vi "G#Object_SendEvent.vi"(0 "reference in":refnum<class "G#Object.lvclass">, 1 "object info extended":T1, 3 "comment":string, 4 "parameters":variant[](array[variant]), 5 "error in (no error)":errorcluster, 6 "G# event type":T3, 7 "send to Desktop Trace Execution":bool=TRUE) -> (19 "error out":errorcluster)   [LabVIEW 2017, in "G#Object.lvclass"]
doc: "Sends object information to the debugger and to the desktop execution trace."
uses:
  G#Object.lvclass
  utils/G#Object_EventType.ctl
  utils/G#Object_ObjectInfoType.ctl
  utils/G#Object_CreateMethod.ctl
  utils/G#Object_Event.ctl
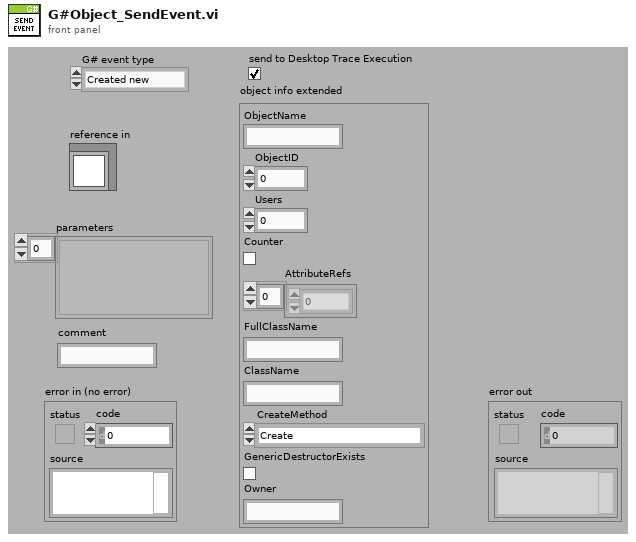
[diagram p1: front panel]
types:
  T1 = typedef "G#Object.lvclass/G#Object_ObjectInfoType.ctl" = cluster{"ObjectName":string, "ObjectID":u32, "Users":i32, "Counter":bool, "AttributeRefs":u32[], "FullClassName":string, "ClassName":string, "CreateMethod":T2, "GenericDestructorExists":bool, "Owner":string}
  T2 = typedef "G#Object.lvclass/G#Object_CreateMethod.ctl" = enum16{"Create", "Create or look up existing", "Look up existing"}
  T3 = typedef "G#Object.lvclass/G#Object_EventType.ctl" = enum16{"Created new", "Looked up existing", "Deleted", "Forced delete", "Not deleted", "Garbage collected", "Cleared", "User", "Error", "External create object", "External create class attributes", "Created class attributes", "Run constructor", "Run constructor done", "Run open method", "Run open method done"}
  T4 = typedef "G#Object.lvclass/G#Object_Event.ctl" = cluster{"EventType":T3, "ObjectInfo":T1, "Ref":refnum<class "G#Object.lvclass">, "Time Stamp":timestamp, "LogText":string, "Parameters":variant[]}
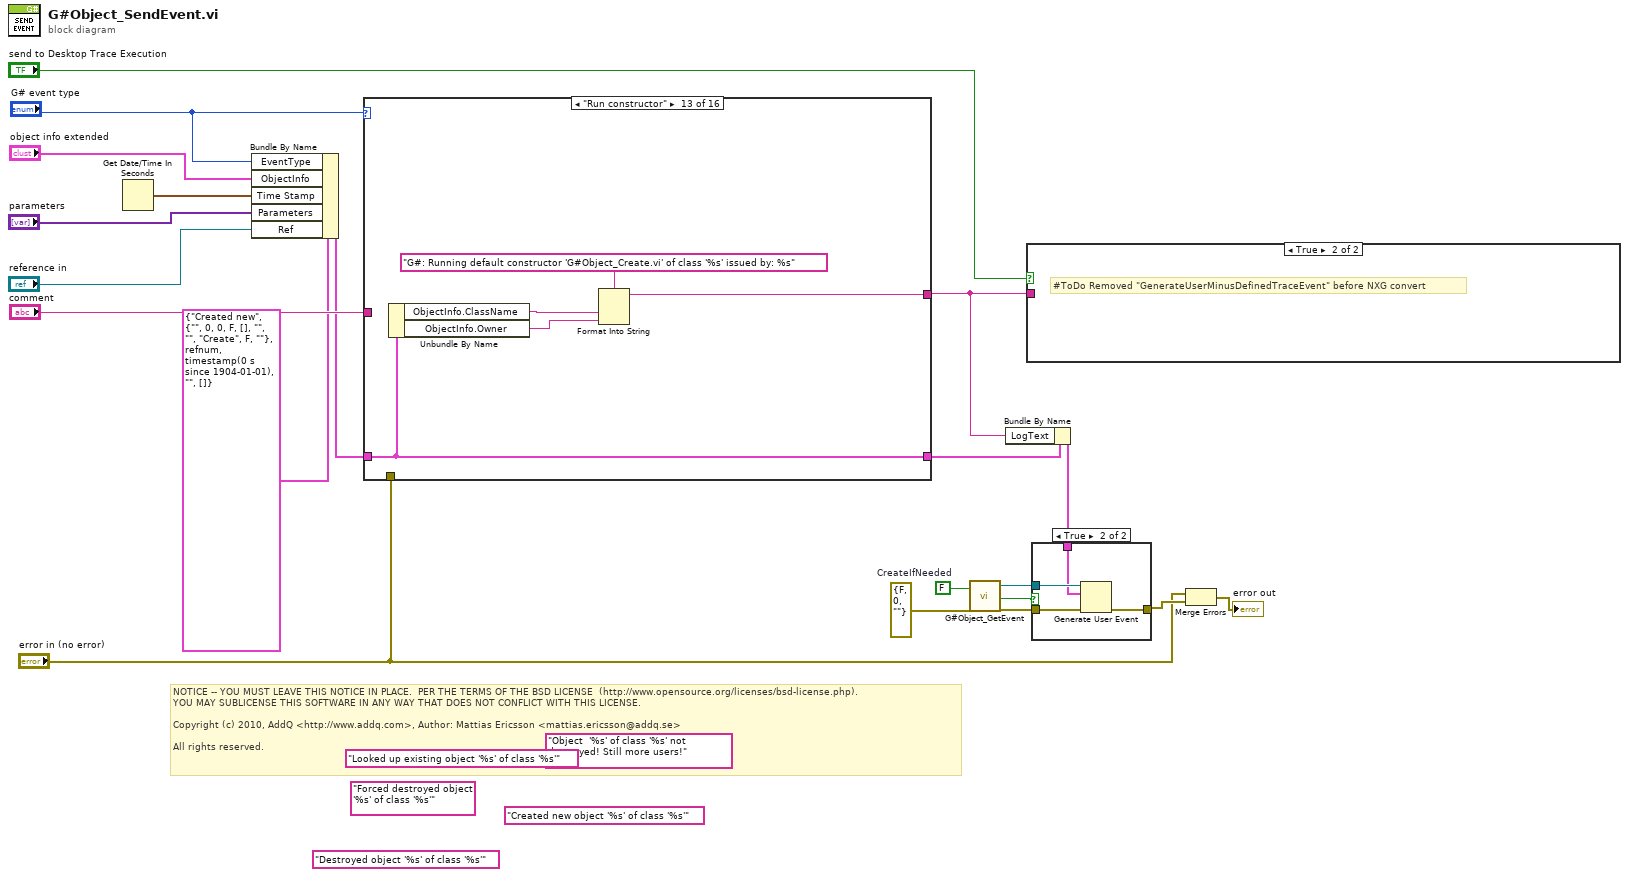
[diagram p0: block diagram]
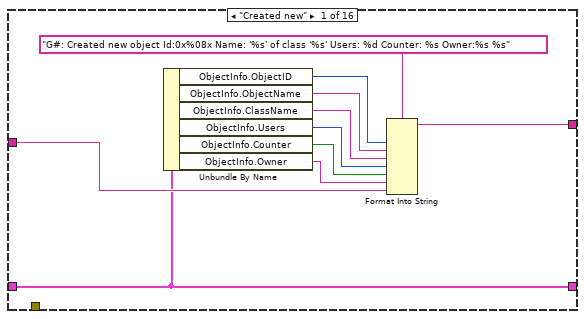
[diagram p4: hidden frame]
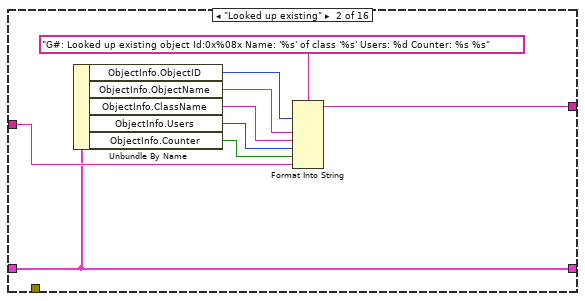
[diagram p5: hidden frame]
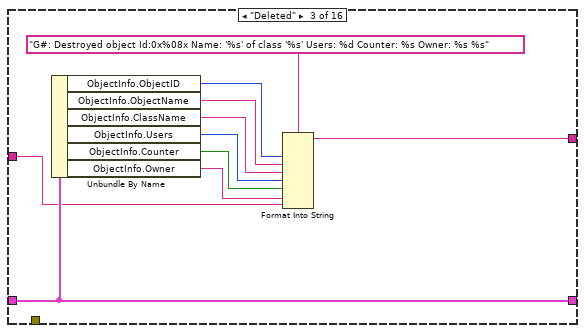
[diagram p6: hidden frame]
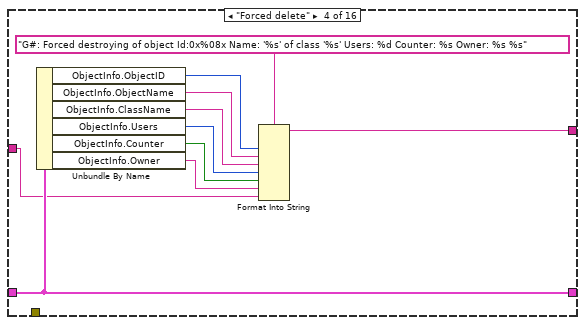
[diagram p7: hidden frame]
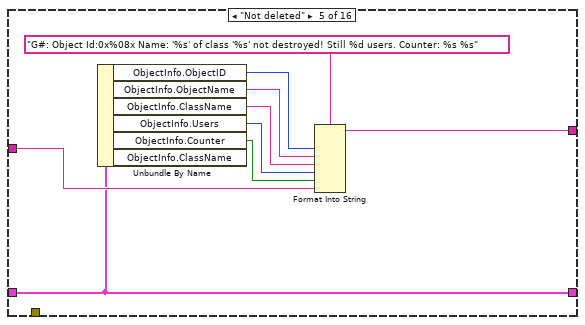
[diagram p8: hidden frame]
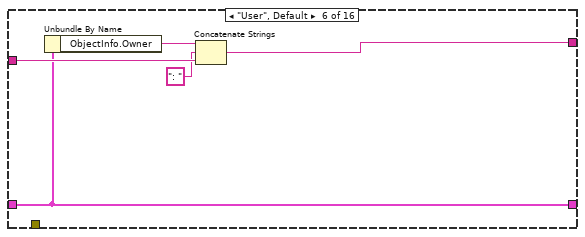
[diagram p9: hidden frame]
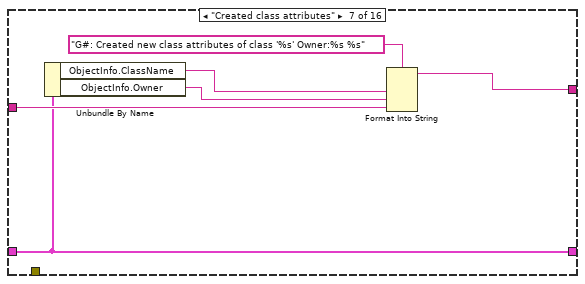
[diagram p10: hidden frame]
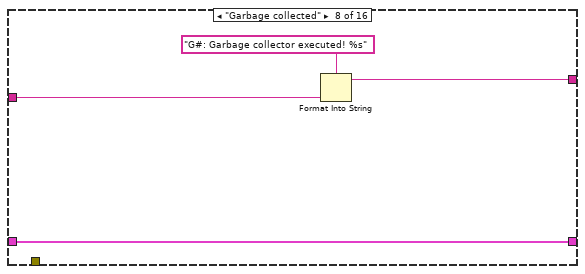
[diagram p11: hidden frame]
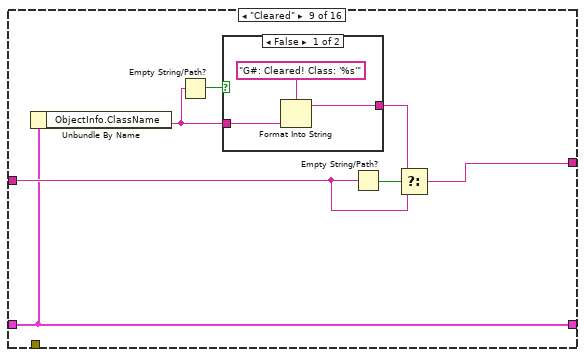
[diagram p12: hidden frame]
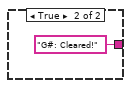
[diagram p13: hidden frame]
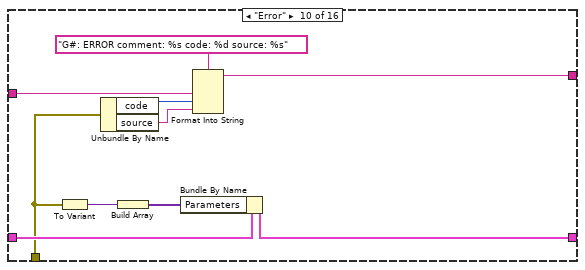
[diagram p14: hidden frame]
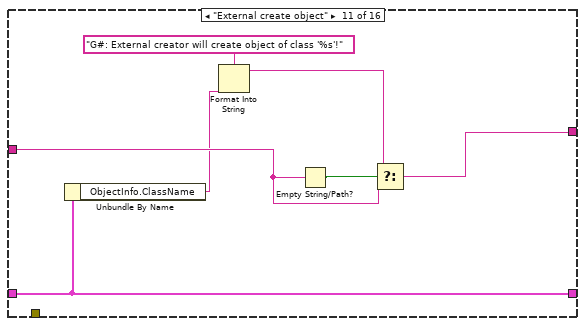
[diagram p15: hidden frame]
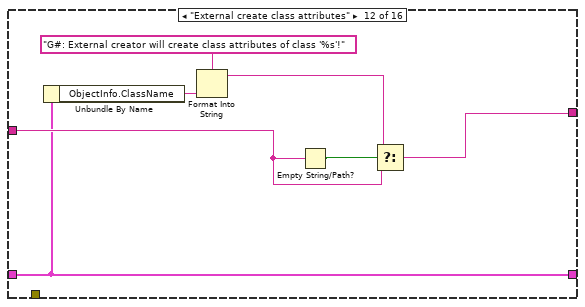
[diagram p16: hidden frame]
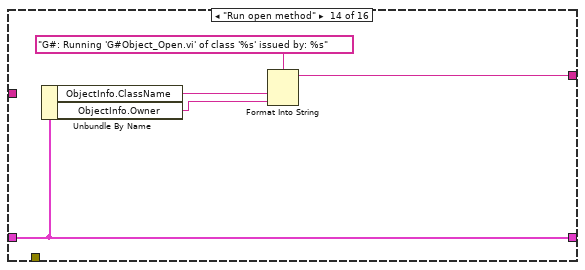
[diagram p17: hidden frame]
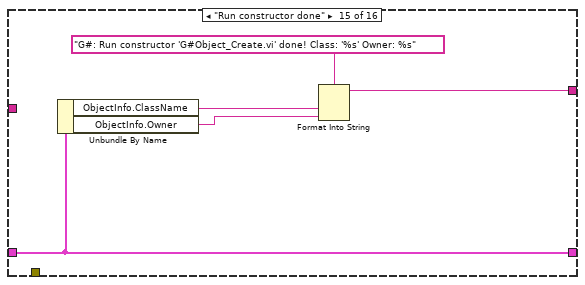
[diagram p18: hidden frame]
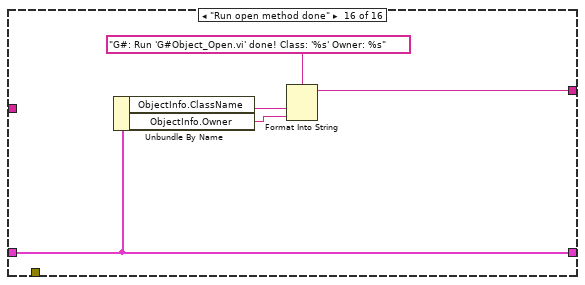
[diagram p19: hidden frame]
diagram:
  w17 = FALSE  # CreateIfNeeded
  (unwired) "Object  '%s' of class '%s' not destroyed! Still more users!"
  (unwired) "Destroyed object '%s' of class '%s'"
  (unwired) "Forced destroyed object '%s' of class '%s'"
  (unwired) "Created new object '%s' of class '%s'"
  (unwired) "Looked up existing object '%s' of class '%s'"
  # "NOTICE -- YOU MUST LEAVE THIS NOTICE IN PLACE.  PER THE TERMS OF THE BSD LICENSE  (http://www.opensource.org/licenses/bsd-license.php).\nYOU MAY SUBLICENSE THIS SOFTWARE IN ANY WAY THAT DOES NOT CONFLICT WITH THIS LICENSE.\n\nCopyright (c) 2010, AddQ <http://www.addq.com>, Author: Mattias Ericsson <mattias.ericsson@addq.se>\n\nAll rights reserved."
  n1 = Get Date/Time In Seconds() -> (seconds since 1Jan1904=w12:timestamp)
  n2 = Bundle By Name(cluster=T4 {"EventType"=enum."Created new", "ObjectInfo"={"ObjectName"="", "ObjectID"=0, "Users"=0, "Counter"=FALSE, "AttributeRefs"=[], "FullClassName"="", "ClassName"="", "CreateMethod"=enum."Create", "GenericDestructorExists"=FALSE, "Owner"=""}, "Ref"=refnum, "Time Stamp"=timestamp(0 s since 1904-01-01), "LogText"="", "Parameters"=[]} ("event data"), "EventType"="G# event type", "ObjectInfo"="object info extended", "Time Stamp"=w12, "Parameters"="parameters", "Ref"="reference in") -> (w4:T4)
  n3 = case shown="\"Run constructor\"" "G# event type" {
    tunnel: [w30 w38 w48 w58 w67 w72 w79 w82 w88 w103 w109 w116 w122 w127 w132 w137] -> w11
    tunnel: "comment" -> [w27 w35 w42 w52 w64 w73 w77 w81 w89 w100 w110 w117 _ _ _ _]
    tunnel: "error in (no error)" -> [_ _ _ _ _ _ _ _ _ w96 _ _ _ _ _ _]
    tunnel: w4 -> [w26 w34 w45 w55 w63 w70 w75 w80 w86 w99 w107 w114 w120 w125 w130 w135]
    tunnel: [w26 w34 w45 w55 w63 w70 w75 w80 w86 w98 w107 w114 w120 w125 w130 w135] -> w3
    frame "Created new" {
      n4 = Unbundle By Name(w26) -> ("ObjectInfo.ObjectID"=w24:u32, "ObjectInfo.ObjectName"=w25:string, "ObjectInfo.ClassName"=w21:string, "ObjectInfo.Users"=w29:i32, "ObjectInfo.Counter"=w22:bool, "ObjectInfo.Owner"=w23:string)
      n5 = Format Into String(format string="G#: Created new object Id:0x%08x Name: '%s' of class '%s' Users: %d Counter: %s Owner:%s %s", w24, w25, w21, w29, w22, w23, w27) -> (resulting string=w30:string)  [unwired: 2 in, 1 out]
    }
    frame "Looked up existing" {
      n6 = Unbundle By Name(w34) -> ("ObjectInfo.ObjectID"=w32:u32, "ObjectInfo.ObjectName"=w33:string, "ObjectInfo.ClassName"=w31:string, "ObjectInfo.Users"=w37:i32, "ObjectInfo.Counter"=w36:bool)
      n7 = Format Into String(format string="G#: Looked up existing object Id:0x%08x Name: '%s' of class '%s' Users: %d Counter: %s %s", w32, w33, w31, w37, w36, w35) -> (resulting string=w38:string)  [unwired: 2 in, 1 out]
    }
    frame "Deleted" {
      n8 = Unbundle By Name(w45) -> ("ObjectInfo.ObjectID"=w43:u32, "ObjectInfo.ObjectName"=w44:string, "ObjectInfo.ClassName"=w40:string, "ObjectInfo.Users"=w47:i32, "ObjectInfo.Counter"=w46:bool, "ObjectInfo.Owner"=w41:string)
      n9 = Format Into String(format string="G#: Destroyed object Id:0x%08x Name: '%s' of class '%s' Users: %d Counter: %s Owner: %s %s", w43, w44, w40, w47, w46, w41, w42) -> (resulting string=w48:string)  [unwired: 2 in, 1 out]
    }
    frame "Forced delete" {
      n10 = Unbundle By Name(w55) -> ("ObjectInfo.ObjectID"=w53:u32, "ObjectInfo.ObjectName"=w54:string, "ObjectInfo.ClassName"=w50:string, "ObjectInfo.Users"=w57:i32, "ObjectInfo.Counter"=w56:bool, "ObjectInfo.Owner"=w51:string)
      n11 = Format Into String(format string="G#: Forced destroying of object Id:0x%08x Name: '%s' of class '%s' Users: %d Counter: %s Owner: %s %s", w53, w54, w50, w57, w56, w51, w52) -> (resulting string=w58:string)  [unwired: 2 in, 1 out]
    }
    frame "Not deleted" {
      n12 = Unbundle By Name(w63) -> ("ObjectInfo.ObjectID"=w61:u32, "ObjectInfo.ObjectName"=w62:string, "ObjectInfo.ClassName"=w60:string, "ObjectInfo.Users"=w66:i32, "ObjectInfo.Counter"=w65:bool)  [unwired: 1 out]
      n13 = Format Into String(format string="G#: Object Id:0x%08x Name: '%s' of class '%s' not destroyed! Still %d users. Counter: %s %s", w61, w62, w60, w66, w65, w64) -> (resulting string=w67:string)  [unwired: 2 in, 1 out]
    }
    frame "User", Default {
      n14 = Unbundle By Name(w70) -> ("ObjectInfo.Owner"=w69:string)
      n15 = Concatenate Strings(w69, ": " ("string"), w73) -> (w72:string)
    }
    frame "Created class attributes" {
      n16 = Unbundle By Name(w75) -> ("ObjectInfo.ClassName"=w76:string, "ObjectInfo.Owner"=w74:string)
      n17 = Format Into String(format string="G#: Created new class attributes of class '%s' Owner:%s %s", w76, w74, w77) -> (resulting string=w79:string)  [unwired: 2 in, 1 out]
    }
    frame "Garbage collected" {
      n18 = Format Into String(format string="G#: Garbage collector executed! %s", w81) -> (resulting string=w82:string)  [unwired: 2 in, 1 out]
    }
    frame "Cleared" {
      n19 = Unbundle By Name(w86) -> ("ObjectInfo.ClassName"=w85:string)
      n20 = Empty String/Path?(string/path=w85) -> (empty?=w84:bool)
      n21 = case shown="False" w84 {
        tunnel: [w92 "G#: Cleared!"] -> w87
        tunnel: w85 -> [w91 _]
        frame False {
          n22 = Format Into String(format string="G#: Cleared! Class: '%s'", w91) -> (resulting string=w92:string)  [unwired: 2 in, 1 out]
        }
        frame True {
        }
      }
      n23 = Empty String/Path?(string/path=w89) -> (empty?=w90:bool)
      n24 = Select(t=w87, s=w90, f=w89) -> (s? t:f=w88:string)
    }
    frame "Error" {
      n25 = To Variant(anything=w96) -> (Variant=w95:variant)
      n26 = Unbundle By Name(w96) -> ("code"=w102:i32, "source"=w101:string)
      n27 = Build Array(w95) -> (w97:variant[])
      n28 = Bundle By Name(cluster=w99, "Parameters"=w97) -> (w98:T4)
      n29 = Format Into String(format string="G#: ERROR comment: %s code: %d source: %s", w100, w102, w101) -> (resulting string=w103:string)  [unwired: 2 in, 1 out]
    }
    frame "External create object" {
      n30 = Unbundle By Name(w107) -> ("ObjectInfo.ClassName"=w106:string)
      n31 = Format Into String(format string="G#: External creator will create object of class '%s'!", w106) -> (resulting string=w105:string)  [unwired: 2 in, 1 out]
      n32 = Empty String/Path?(string/path=w110) -> (empty?=w111:bool)
      n33 = Select(t=w105, s=w111, f=w110) -> (s? t:f=w109:string)
    }
    frame "External create class attributes" {
      n34 = Unbundle By Name(w114) -> ("ObjectInfo.ClassName"=w113:string)
      n35 = Format Into String(format string="G#: External creator will create class attributes of class '%s'!", w113) -> (resulting string=w112:string)  [unwired: 2 in, 1 out]
      n36 = Empty String/Path?(string/path=w117) -> (empty?=w118:bool)
      n37 = Select(t=w112, s=w118, f=w117) -> (s? t:f=w116:string)
    }
    frame "Run constructor" {
      n38 = Unbundle By Name(w120) -> ("ObjectInfo.ClassName"=w121:string, "ObjectInfo.Owner"=w119:string)
      n39 = Format Into String(format string="G#: Running default constructor 'G#Object_Create.vi' of class '%s' issued by: %s", w121, w119) -> (resulting string=w122:string)  [unwired: 2 in, 1 out]
    }
    frame "Run open method" {
      n40 = Unbundle By Name(w125) -> ("ObjectInfo.ClassName"=w126:string, "ObjectInfo.Owner"=w124:string)
      n41 = Format Into String(format string="G#: Running 'G#Object_Open.vi' of class '%s' issued by: %s", w126, w124) -> (resulting string=w127:string)  [unwired: 2 in, 1 out]
    }
    frame "Run constructor done" {
      n42 = Unbundle By Name(w130) -> ("ObjectInfo.ClassName"=w131:string, "ObjectInfo.Owner"=w129:string)
      n43 = Format Into String(format string="G#: Run constructor 'G#Object_Create.vi' done! Class: '%s' Owner: %s" ("comment"), w131, w129) -> (resulting string=w132:string)  [unwired: 2 in, 1 out]
    }
    frame "Run open method done" {
      n44 = Unbundle By Name(w135) -> ("ObjectInfo.ClassName"=w136:string, "ObjectInfo.Owner"=w134:string)
      n45 = Format Into String(format string="G#: Run 'G#Object_Open.vi' done! Class: '%s' Owner: %s" ("comment"), w136, w134) -> (resulting string=w137:string)  [unwired: 2 in, 1 out]
    }
  }
  n46 = call "G#Object_GetEvent.vi"("create if needed (T)"=w17, "error in (no error)"=errorcluster {"status"=FALSE, "code"=0, "source"=""}) -> ("G# event"=w14:refnum<user-event>, "valid"=w10:bool, "error out"=w15:errorcluster)  [unwired: 13 in, 2 out]
  n47 = Bundle By Name(cluster=w3, "LogText"=w11) -> (w13:T4)
  n48 = case shown="True" "send to Desktop Trace Execution" {
    tunnel: w11 -> [_ _]
    frame False {
    }
    frame True {
      # "#ToDo Removed \"GenerateUserMinusDefinedTraceEvent\" before NXG convert"
    }
  }
  n49 = case shown="True" w10 {
    tunnel: w15 -> [w139 w143]
    tunnel: [w139 w142] -> w8
    tunnel: w14 -> [_ w141]
    tunnel: w13 -> [_ w140]
    frame False {
    }
    frame True {
      n50 = Generate User Event(user event=w141, event data cluster=w140, error in=w143) -> (error out=w142:errorcluster)  [unwired: 1 in, 1 out]
    }
  }
  n51 = Merge Errors("error in (no error)", w8) -> (→"error out":errorcluster)
